vi "konverter.vi"() -> ()   [LabVIEW 2010]
panel:
  out "Text":string
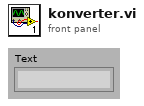
[diagram p1: front panel]
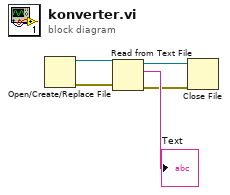
[diagram p0: block diagram]
diagram:
  n1 = Open/Create/Replace File() -> (refnum out=w5:refnum<file>, error out=w4:errorcluster)  [unwired: 6 in, 1 out]
  n2 = Read from Text File(file (use dialog)=w5, error in=w4) -> (refnum out=w2:refnum<file>, text=→"Text":string, error out=w1:errorcluster)  [unwired: 2 in, 1 out]
  n3 = Close File(refnum=w2, error in=w1) -> ()  [unwired: 2 out]
